vi "Test_Multiple_Panel.vi"() -> ()   [LabVIEW 2021]
panel:
  out "Loading#":i32
  in  "Loading":bool
  in  "Exit":bool
  in  "Test Panel#":i32=5
  in  "Time Target (s)":dbl=5.0 format="%.0p"
  in  "System_Delay(s)":dbl=0.01 format="%.0p"
  in  "State_Interval_Time(s)":dbl=0.01 format="%.0p"
  in  "State#":i32=1000
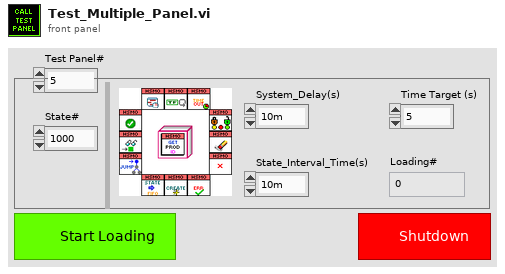
[diagram p1: front panel]
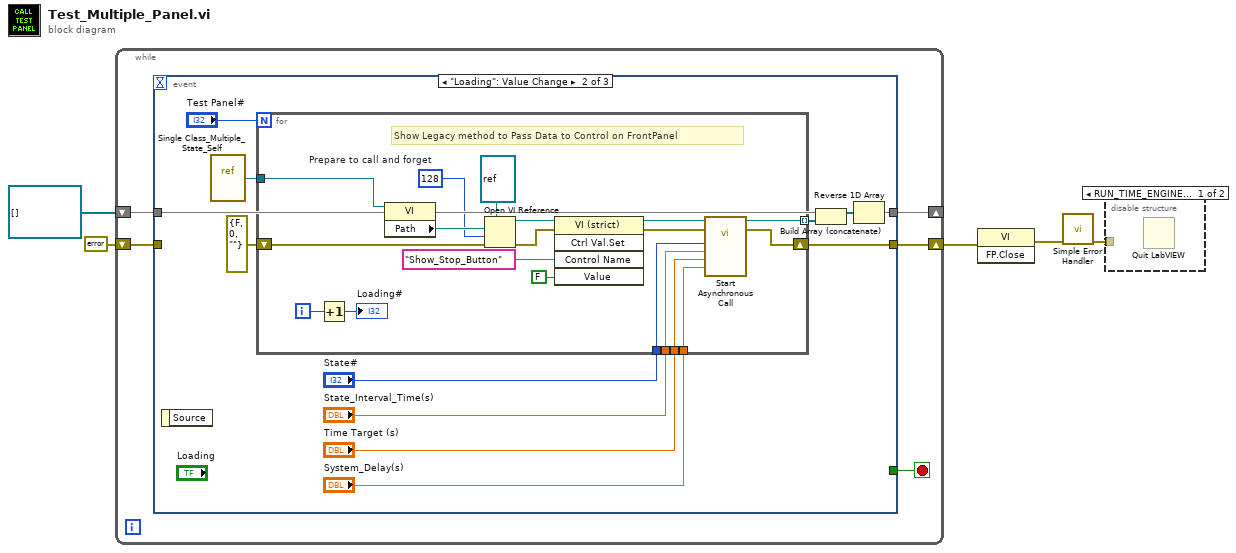
[diagram p0: block diagram]
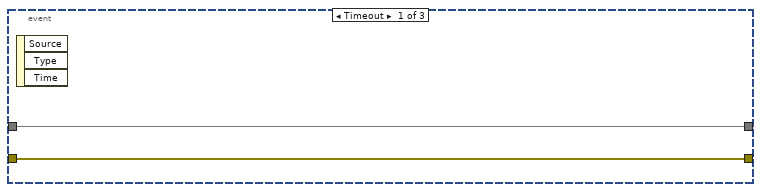
[diagram p3: hidden frame]
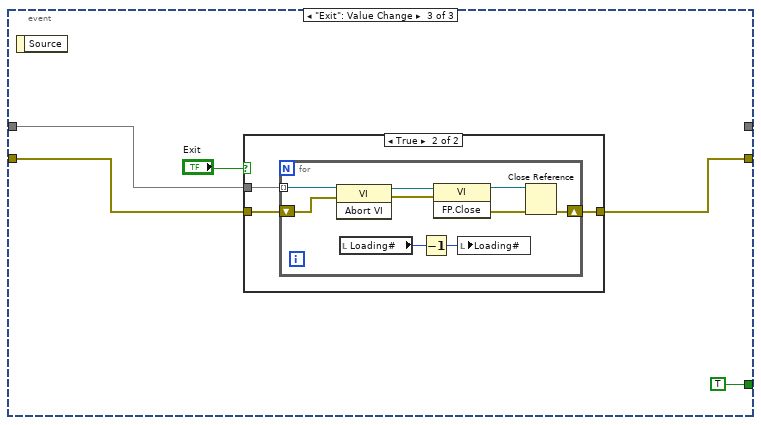
[diagram p4: hidden frame]
diagram:
  n1 = while {
    shift-right: [w10] -> _
    shift-left: refnum<vi>[] [] -> [w8]
    shift-right: [w9] -> w3
    shift-left: errorcluster {"status"=FALSE, "code"=0, "source"=""} ("error out") -> [w7]
    stop <- w6 stop-if-true
    n2 = event shown="[1] \"Loading\": Value Change" {
      selector: _ -> [_ _ _]
      dyn-events: _ -> [_ _ _]
      timeout: _ -> [_ _ _]
      tunnel: [w12 w13 _] -> w10
      tunnel: [w11 w16 w45] -> w9
      tunnel: w8 -> [w12 w14 w47]
      tunnel: w7 -> [w11 _ w46]
      tunnel: [_ _ TRUE] -> w6
      event Timeout {
        n3 = event-data() -> ()  [unwired: 1 in, 3 out]
      }
      event "Loading": Value Change {
        n4 = event-data() -> ()  [unwired: 1 in, 1 out]
        n5 = vi-ref "Single Class_Multiple_State_Self.vi"() -> (w20:refnum<vi>)
        n6 = for {
          N: "Test Panel#" -> [_]
          shift-right: [w30] -> w16
          shift-left: errorcluster {"status"=FALSE, "code"=0, "source"=""} ("error out") -> [w32]
          tunnel: w20 -> [w41]
          tunnel: "State#" -> [w28]
          tunnel: "State_Interval_Time(s)" -> [w27]
          tunnel: "System_Delay(s)" -> [w25]
          tunnel: "Time Target (s)" -> [w26]
          tunnel: [w31] -> w17 mode=indexing
          i -> [w35]
          w40 = 128  # Prepare to call and forget
          # "Show Legacy method to Pass Data to Control on FrontPanel"
          n7 = Increment(x=w35) -> (x+1=→"Loading#":i32)
          n8 = property class="VI"(reference=w41) -> ("Path"=w43:path)  [unwired: 1 in, 2 out]
          n9 = Open VI Reference(type specifier VI Refnum (for type only)=refnum<vi> refnum, vi path=w43, options=w40, error in (no error)=w32) -> (vi reference=w33:refnum<vi>, error out=w38:errorcluster)  [unwired: 2 in]
          n10 = invoke class="VI (strict)" method="Ctrl Val.Set"(reference=w33, error in=w38, "Control Name"="Show_Stop_Button", "Value"=FALSE) -> (reference out=w29:refnum<vi>, error out=w39:errorcluster)  [unwired: 1 in, 3 out]
          n11 = call-by-ref "Start Asynchronous Call"(reference=w29, error in=w39, "State#"=w28, "State_Interval_Time(s)"=w27, "Time Target (s)"=w26, "System_Delay(s)"=w25) -> (reference out=w31:refnum<vi>, error out=w30:errorcluster)  [unwired: 5 in]
        }
        n12 = Build Array (concatenate)(w14, w17) -> (w15:refnum<vi>[])
        n13 = Reverse 1D Array(array=w15) -> (reversed array=w13:refnum<vi>[])
      }
      event "Exit": Value Change {
        n14 = event-data() -> ()  [unwired: 1 in, 1 out]
        n15 = case shown="True" "Exit" {
          tunnel: w47 -> [_ w52]
          tunnel: w46 -> [w49 w51]
          tunnel: [w49 w50] -> w45
          frame False {
          }
          frame True {
            n16 = for {
              tunnel: w52 -> [w56] mode=indexing
              shift-right: [w57] -> w50
              shift-left: w51 -> [w53]
              n17 = invoke class="VI" method="Abort VI"(reference=w56, error in=w53) -> (reference out=w55:refnum<vi>, error out=w54:errorcluster)  [unwired: 1 in, 1 out]
              n18 = local read "Loading#"() -> (w59:i32)
              n19 = Decrement(x=w59) -> (x-1=w58:i32)
              n20 = invoke class="VI" method="FP.Close"(reference=w55, error in=w54) -> (reference out=w61:refnum<vi>, error out=w60:errorcluster)  [unwired: 1 in, 1 out]
              n21 = local write "Loading#"(w58) -> ()
              n22 = Close Reference(reference=w61, error in (no error)=w60) -> (error out=w57:errorcluster)
            }
          }
        }
      }
    }
  }
  n23 = invoke class="VI" method="FP.Close"(error in=w3) -> (error out=w5:errorcluster)  [unwired: 2 in, 2 out]
  n24 = call <vilib>:"Simple Error Handler.vi"("error in (no error)"=w5) -> ("error out"=w2:errorcluster)  [unwired: 4 in, 4 out]
  n25 = disable-structure shown="RUN_TIME_ENGINE==True" {
    disable-tunnel: w2 -> [_ _]
    frame condition #0 {
      n26 = Quit LabVIEW() -> ()  [unwired: 1 in]
    }
    frame condition #1 (active) {
    }
  }
